vi "Append Gas Inspection Waypoint.vi"(0 "Waypoint Array In":T1[](array[typedef]), 5 "Lat":sgl, 7 "Lon":sgl, 9 "Altitude (m)":sgl, 11 "Error In":errorcluster, 12 "Inspection altitude (m)":sgl=10.0, 13 "Pump time (sec)":sgl=5.0) -> (4 "appended array":T1[](array[typedef]), 15 "Error Out":errorcluster)   [LabVIEW 2014]
uses:
  Controls/Mission Planning Controls/MAVLINK Mission Item.ctl
  Controls/MAVLINK Mav Frame.ctl
  Commands/Mission Planning/MISSION_ITEM SubVI/MISSION_ITEM Loiter (Time).vi
  Commands/Mission Planning/MISSION_ITEM SubVI/MISSION_ITEM Condition YAW.vi
  Commands/Mission Planning/MISSION_ITEM SubVI/MISSION_ITEM Set Servo Repeat.vi
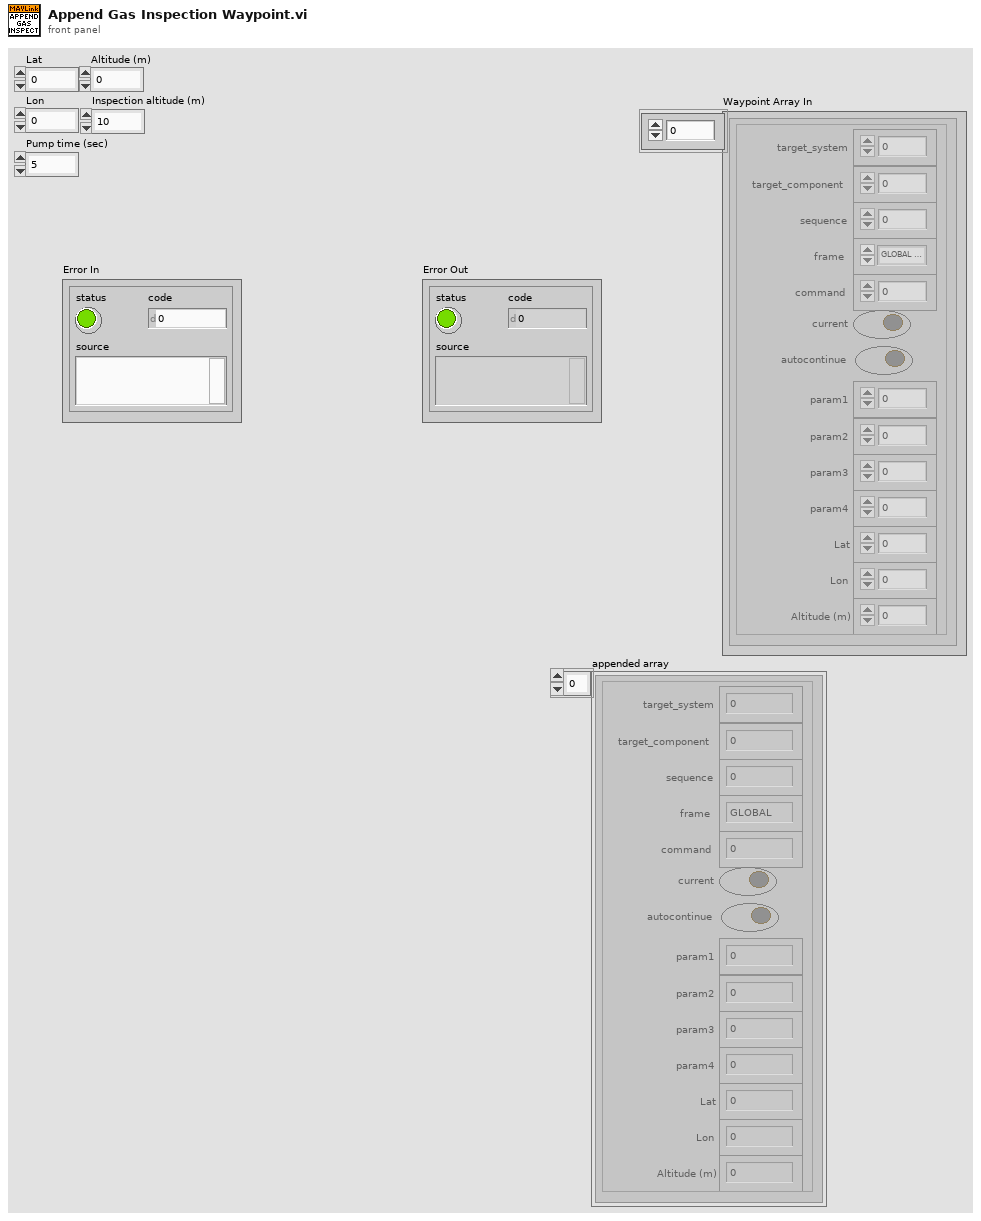
[diagram p1: front panel]
types:
  T1 = typedef "MAVLINK Mission Item.ctl" = cluster{"target_system":u8, "target_component":u8, "sequence":u16, "frame":T2, "command":u16, "current":bool, "autocontinue":bool, "param1":sgl, "param2":sgl, "param3":sgl, "param4":sgl, "Lat":sgl, "Lon":sgl, "Altitude (m)":sgl}
  T2 = typedef "MAVLINK Mav Frame.ctl" = enum8{"GLOBAL", "LOCAL NED", "MISSION", "GLOBAL RELATIVE ALT", "LOCAL ENU", "GLOBAL INT", "GLOBAL RELATIVE ALT INT", "LOCAL OFFSET NED", "BODY NED", "BODY OFFSET NED", "GLOBAL TERRAIN ALT", "GLOBAL TERRAIN ALT INT"}
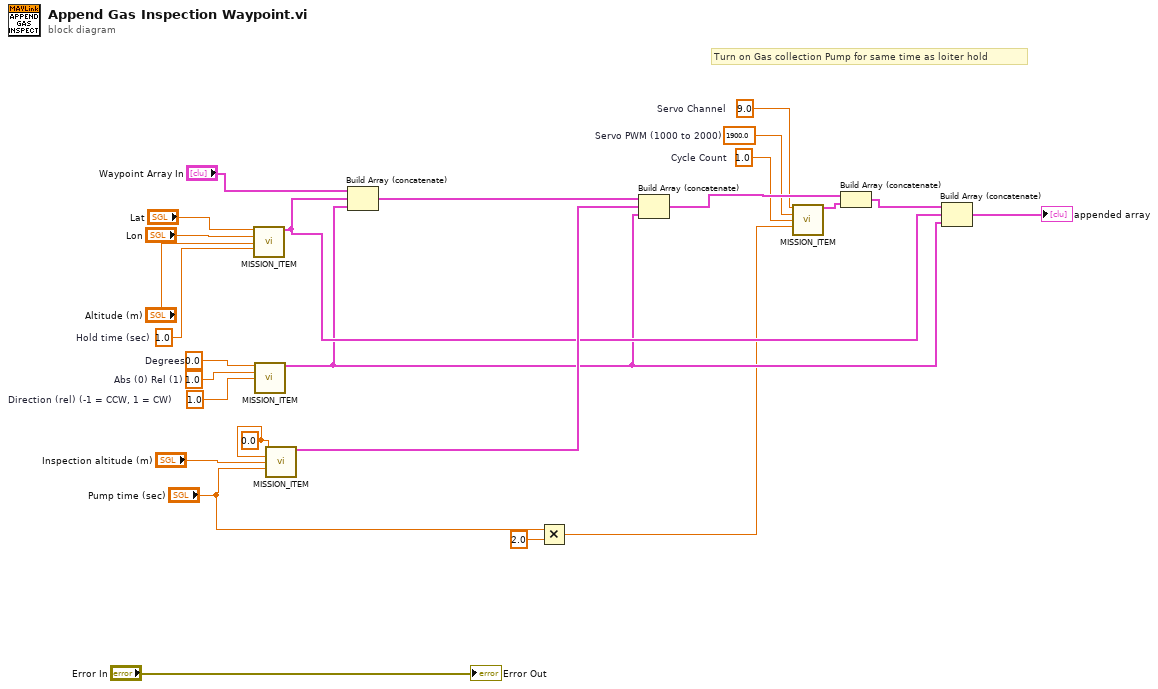
[diagram p0: block diagram]
diagram:
  w4 = sgl 1.0  # Cycle Count
  w5 = sgl 1900.0  # Servo PWM (1000 to 2000)
  w6 = sgl 9.0  # Servo Channel
  w16 = sgl 1.0  # Direction (rel) (-1 = CCW, 1 = CW)
  w17 = sgl 1.0  # Abs (0) Rel (1)
  w18 = sgl 0.0  # Degrees
  w19 = sgl 0.0 ("Lat")
  w22 = sgl 1.0  # Hold time (sec)
  # "Turn on Gas collection Pump for same time as loiter hold"
  n1 = call-poly "MISSION_ITEM.vi"("Lat"="Lat", "Lon"="Lon", "Altitude (m)"="Altitude (m)", "Loiter time (sec)"=w22) -> ("Mission Item"=w11:T1)  [unwired: 11 in]
  n2 = call-poly "MISSION_ITEM.vi"("Degrees"=w18, "Abs (0) Rel (1)"=w17, "Direction (rel) (-1 = CCW, 1 = CW)"=w16) -> ("Mission Item"=w10:T1)  [unwired: 12 in]
  n3 = call-poly "MISSION_ITEM.vi"("Lat"=w19, "Lon"=w19, "Altitude (m)"="Inspection altitude (m)", "Loiter time (sec)"="Pump time (sec)") -> ("Mission Item"=w14:T1)  [unwired: 11 in]
  n4 = Build Array (concatenate)("Waypoint Array In", w11, w10) -> (w7:T1[])
  n5 = Multiply(x="Pump time (sec)", y=sgl 2.0) -> (x*y=w1:sgl)
  n6 = Build Array (concatenate)(w7, w14, w10) -> (w13:T1[])
  n7 = call-poly "MISSION_ITEM.vi"("Servo Channel"=w6, "Servo PWM (1000 to 2000)"=w5, "Cycle Count"=w4, "Cycle Time (s)"=w1) -> ("Mission Item"=w8:T1)  [unwired: 11 in]
  n8 = Build Array (concatenate)(w13, w8) -> (w12:T1[])
  n9 = Build Array (concatenate)(w12, w11, w10) -> (→"appended array":T1[])
  "Error Out" <- "Error In"
